vi "EIP Write Tags.vi"(4 "Previous Values buffer":cluster{"Tag Values":dbl[]}[](array[cluster]), 6 "Tag Data":T3[](array[typedef]) {"Device Reference" format="%.0x"}, 7 "Device Settings":T2, 8 "error in":errorcluster, 9 "Session In":T1, 10 "Device Inputs In":dbl[](array[numeric]), 11 "Device Inputs FIFO":refnum<k33>) -> (0 "error out":errorcluster, 1 "Session Out":T1, 2 "Device Inputs Out":dbl[](array[numeric]))   [LabVIEW 2011, in "Ethernet IP Custom Device Custom Device.lvlib"]
uses:
  Ethernet IP Custom Device Custom Device.lvlib
  EIP Tag Information.ctl
  <vilib>/NI Veristand/Custom Device API/Custom Device Item Info.ctl
  <vilib>/NI Veristand/Custom Device API/Custom Device Item Ref.ctl
  L5K Data Types.ctl
  EIP Device Settings.ctl
  <vilib>/ethernetip/ethernetip.llb/ethernetip.ctl
  <vilib>/ethernetip/ethernetip.llb/EthernetIP Tag Write SINT.vi
  <vilib>/ethernetip/ethernetip.llb/EthernetIP Tag Write INT.vi
  <vilib>/ethernetip/ethernetip.llb/EthernetIP Tag Write DINT.vi
  <vilib>/ethernetip/ethernetip.llb/EthernetIP Tag Write REAL.vi
  <vilib>/ethernetip/ethernetip.llb/EthernetIP Tag Write BOOL.vi
  <vilib>/ethernetip/ethernetip.lvlib
  <vilib>/NI Veristand/Custom Device API/Custom Device API.lvlib
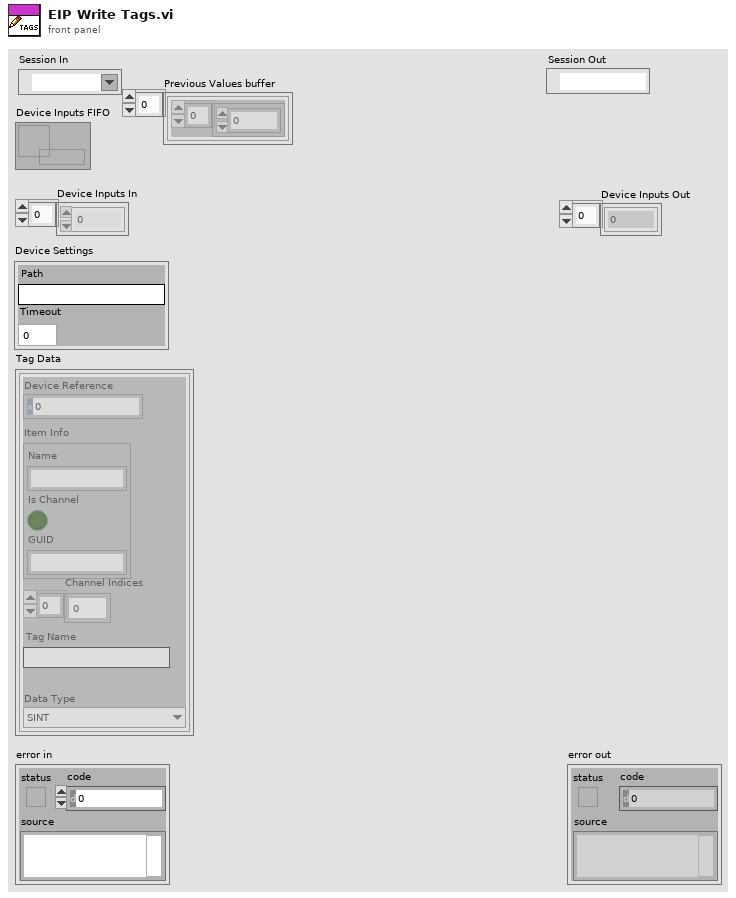
[diagram p1: front panel]
types:
  T1 = typedef "ethernetip.lvlib/ethernetip.ctl" = refnum<k21>
  T2 = typedef "Ethernet IP Custom Device Custom Device.lvlib/EIP Device Settings.ctl" = cluster{"Path":string, "Timeout":i32}
  T3 = typedef "Ethernet IP Custom Device Custom Device.lvlib/EIP Tag Information.ctl" = cluster{"Item Info":T4, "Device Reference":T5, "Channel Indices":i32[], "Tag Name":string, "Data Type":T6}
  T4 = typedef "Custom Device API.lvlib/Custom Device Item Info.ctl" = cluster{"Name":string, "Is Channel":bool, "GUID":string}
  T5 = typedef "Custom Device API.lvlib/Custom Device Item Ref.ctl" = u64
  T6 = typedef "Ethernet IP Custom Device Custom Device.lvlib/L5K Data Types.ctl" = enum16{"SINT", "INT", "DINT", "REAL", "BOOL"}
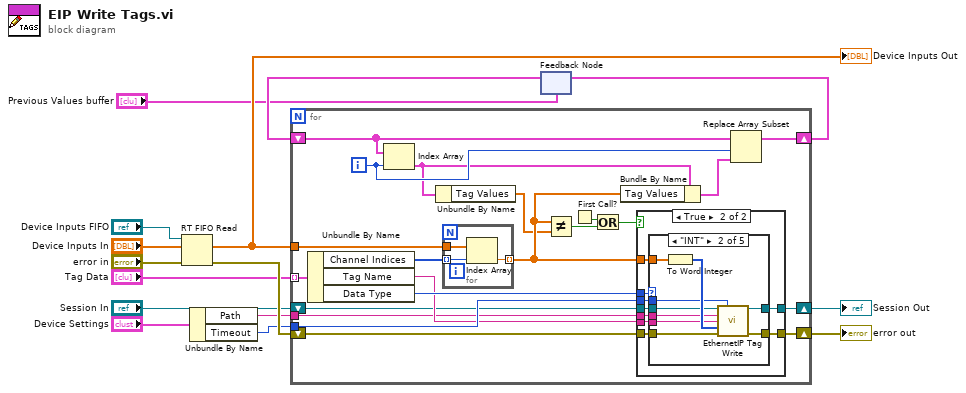
[diagram p0: block diagram]
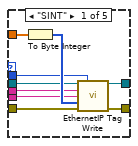
[diagram p3: hidden frame]
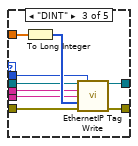
[diagram p4: hidden frame]
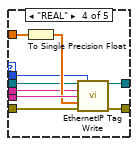
[diagram p5: hidden frame]
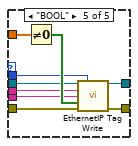
[diagram p6: hidden frame]
diagram:
  n1 = RT FIFO Read(0:"Device Inputs FIFO", 1:"Device Inputs In", 3:"error in") -> (9:w7:dbl[], 11:w12:errorcluster)  [unwired: 1 in, 3 out]
  "Device Inputs Out" <- w7
  n2 = Unbundle By Name("Device Settings") -> ("Path"=w10:string, "Timeout"=w9:i32)
  n3 = feedback #1("Previous Values buffer") -> (w3:cluster{"Tag Values":dbl[]}[])
  n4 = for {
    tunnel: w7 -> [w35]
    shift-right: [w31] -> w6
    shift-left: w12 -> [w32]
    tunnel: w10 -> [w28]
    tunnel: w9 -> [w30]
    tunnel: "Tag Data" -> [w36] mode=indexing
    shift-right: [w26] -> w4
    shift-left: "Session In" -> [w27]
    shift-right: [w21] -> w1
    shift-left: w3 -> [w25]
    i -> [w24]
    n5 = Unbundle By Name(w36) -> ("Channel Indices"=w34:i32[], "Tag Name"=w29:string, "Data Type"=w33:T6)
    n6 = Index Array(array=w25, index=w24) -> (element=w23:cluster{"Tag Values":dbl[]})
    n7 = Unbundle By Name(w23) -> ("Tag Values"=w19:dbl[])
    n8 = for {
      tunnel: w35 -> [w93]
      tunnel: w34 -> [w95] mode=indexing
      tunnel: [w94] -> w20 mode=indexing
      n9 = Index Array(array=w93, index=w95) -> (element=w94:dbl)
    }
    n10 = Not Equal?(x=w20, y=w19) -> (x != y?=w18:bool)
    n11 = First Call?() -> (First Call?: T/F=w17:bool)
    n12 = Or(x=w17, y=w18) -> (x .or. y?=w16:bool)
    n13 = Bundle By Name(cluster=w23, "Tag Values"=w20) -> (w22:cluster{"Tag Values":dbl[]})
    n14 = case shown="True" w16 {
      tunnel: w33 -> [_ w47]
      tunnel: w32 -> [w37 w46]
      tunnel: [w37 w45] -> w31
      tunnel: w30 -> [_ w44]
      tunnel: w29 -> [_ w43]
      tunnel: w28 -> [_ w42]
      tunnel: w27 -> [w38 w41]
      tunnel: [w38 w40] -> w26
      tunnel: w20 -> [_ w39]
      frame False {
      }
      frame True {
        n15 = case shown="\"INT\"" w47 {
          tunnel: w43 -> [w54 w63 w72 w83 w90]
          tunnel: w39 -> [w56 w65 w74 w82 w92]
          tunnel: w42 -> [w51 w59 w69 w78 w87]
          tunnel: w44 -> [w50 w60 w68 w77 w86]
          tunnel: w46 -> [w53 w62 w71 w80 w89]
          tunnel: [w52 w61 w70 w79 w88] -> w45
          tunnel: w41 -> [w48 w57 w67 w76 w84]
          tunnel: [w49 w58 w66 w75 w85] -> w40
          frame "SINT" {
            n16 = To Byte Integer(number=w56) -> (8bit integer=w55:i8[])
            n17 = call-poly <vilib>:"EthernetIP Tag Write.vi"("Session in"=w48, "Timeout (ms)"=w50, "Network Path"=w51, "Tag Name"=w54, "Data"=w55, "error in"=w53) -> ("Session out"=w49:T1, "error out"=w52:errorcluster)  [unwired: 8 in]
          }
          frame "INT" {
            n18 = To Word Integer(number=w65) -> (16bit integer=w64:i16[])
            n19 = call-poly <vilib>:"EthernetIP Tag Write.vi"("Session in"=w57, "Timeout (ms)"=w60, "Network Path"=w59, "Tag Name"=w63, "Data"=w64, "error in"=w62) -> ("Session out"=w58:T1, "error out"=w61:errorcluster)  [unwired: 8 in]
          }
          frame "DINT" {
            n20 = To Long Integer(number=w74) -> (32bit integer=w73:i32[])
            n21 = call-poly <vilib>:"EthernetIP Tag Write.vi"("Session in"=w67, "Timeout (ms)"=w68, "Network Path"=w69, "Tag Name"=w72, "Data"=w73, "error in"=w71) -> ("Session out"=w66:T1, "error out"=w70:errorcluster)  [unwired: 8 in]
          }
          frame "REAL" {
            n22 = To Single Precision Float(number=w82) -> (single precision float=w81:sgl[])
            n23 = call-poly <vilib>:"EthernetIP Tag Write.vi"("Session in"=w76, "Timeout (ms)"=w77, "Network Path"=w78, "Tag Name"=w83, "Data"=w81, "error in"=w80) -> ("Session out"=w75:T1, "error out"=w79:errorcluster)  [unwired: 8 in]
          }
          frame "BOOL" {
            n24 = Not Equal To 0?(x=w92) -> (x != 0?=w91:bool[])
            n25 = call-poly <vilib>:"EthernetIP Tag Write.vi"("Session in"=w84, "Timeout (ms)"=w86, "Network Path"=w87, "Tag Name"=w90, "Data"=w91, "error in"=w89) -> ("Session out"=w85:T1, "error out"=w88:errorcluster)  [unwired: 8 in]
          }
        }
      }
    }
    n26 = Replace Array Subset(array=w25, new element=w22, index=w24) -> (w21:cluster{"Tag Values":dbl[]}[])
  }
  "error out" <- w6
  "Session Out" <- w4
  n27 = feedback-in #1(w1) -> ()
